vi "Superimpose Display X And A B Mode.vi"(6 "Superimpose Limit (F:Off)":bool, 8 "error in (no error)":errorcluster, 9 "SuperimposeDispDataB(F:Off)":bool, 10 "SuperimposeDispDataA(F:Off)":bool, 11 "VISA resource name":refnum<visa-resource-name>) -> (0 "error out":errorcluster, 3 "VISA resource name out":refnum<visa-resource-name>)   [LabVIEW 2010, in "Agilent 4194.lvlib"]
doc: "This function is used for compare old and new data on instrument's display effective for X - A&B.\n\nNotes:\n\n(1) This function is valid for X - A&B setting only."
uses:
  <instrlib>/Agilent 4194/Agilent 4194.lvlib
panel:
  # "On\nOff"
  # "On\nOff"
  # "On\nOff"
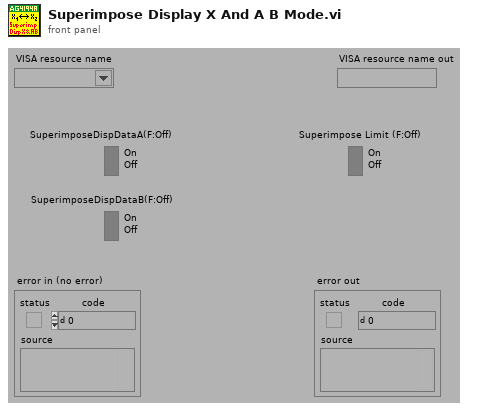
[diagram p1: front panel]
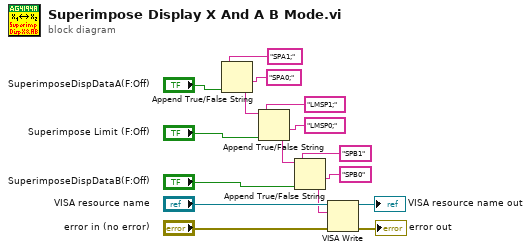
[diagram p0: block diagram]
diagram:
  n1 = Append True/False String(1:"SuperimposeDispDataA(F:Off)", 2:"SPA0;", 3:"SPA1;") -> (0:w6:string)  [unwired: 1 in]
  n2 = Append True/False String(1:"Superimpose Limit (F:Off)", 2:"LMSP0;", 3:"LMSP1;", 4:w6) -> (0:w2:string)
  n3 = Append True/False String(1:"SuperimposeDispDataB(F:Off)", 2:"SPB0", 3:"SPB1", 4:w2) -> (0:w1:string)
  n4 = VISA Write(VISA resource name="VISA resource name", write buffer=w1, error in (no error)="error in (no error)") -> (VISA resource name out=→"VISA resource name out":refnum<visa-resource-name>, error out=→"error out":errorcluster)  [unwired: 1 out]
